vi "GenerateUntriggeredStimulus.vi"(8 "error in (no error)":errorcluster, 11 "HeadandTailRailswithDelay in":refnum<class "HeadandTailRailswithDelay.lvclass">) -> (0 "error out":errorcluster, 2 "UntriggeredStimulusOut":sgl[][](array[numeric]), 3 "HeadandTailRailswithDelay out":refnum<class "HeadandTailRailswithDelay.lvclass">)   [LabVIEW 2019, in "HeadandTailRailswithDelay.lvclass"]
uses:
  HeadandTailRailswithDelay.lvclass
  HeadandTailRailswithDelay.lvclass/HeadandTailRailswithDelay.ctl
  ParametersGlobal.vi
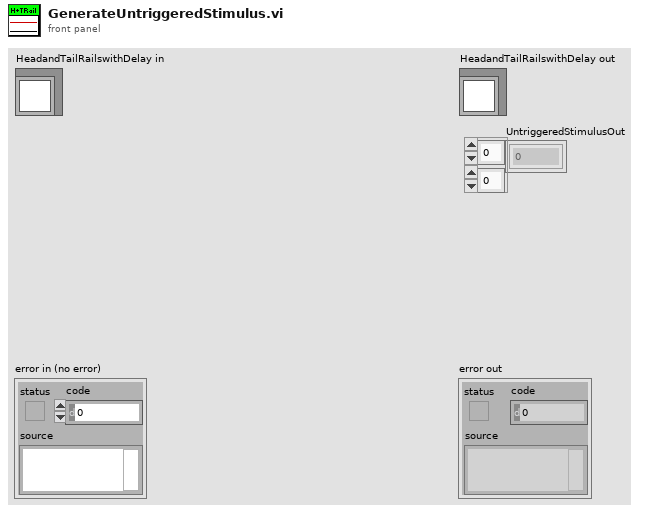
[diagram p1: front panel]
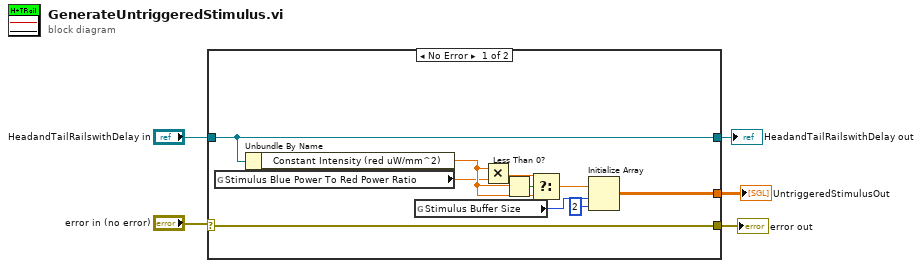
[diagram p0: block diagram]
diagram:
  n1 = case shown="No Error" "error in (no error)" {
    selector: "error in (no error)" -> [w15 w17]
    tunnel: [w15 w17] -> w2
    tunnel: [w14 w16] -> w3
    tunnel: "HeadandTailRailswithDelay in" -> [w14 w16]
    tunnel: [w8 _] -> w1
    frame No Error {
      n2 = global read "ParametersGlobal.vi" "Stimulus Blue Power To Red Power Ratio"() -> (w10:sgl)
      n3 = Unbundle By Name(w14) -> ("Constant Intensity (red uW/mm^2)"=w11:sgl)
      n4 = global read "ParametersGlobal.vi" "Stimulus Buffer Size"() -> (w7:i32)
      n5 = Multiply(x=w11, y=w10) -> (x*y=w13:sgl)
      n6 = Less Than 0?(x=w11) -> (x < 0?=w12:bool)
      n7 = Select(t=w13, s=w12, f=w11) -> (s? t:f=w9:sgl)
      n8 = Initialize Array(w9, w7, 2 ("dimension size")) -> (w8:sgl[][])
    }
    frame Error {
    }
  }
  "error out" <- w2
  "HeadandTailRailswithDelay out" <- w3
  "UntriggeredStimulusOut" <- w1
